vi "remove void rows.vi"(8 "error in":errorcluster, 11 "Group run list input":string[][](array[string])) -> (0 "error out":errorcluster, 3 "Group run list":string[][](array[string]))   [LabVIEW 2016]
doc: "This vi removes any empty spots from the run order."
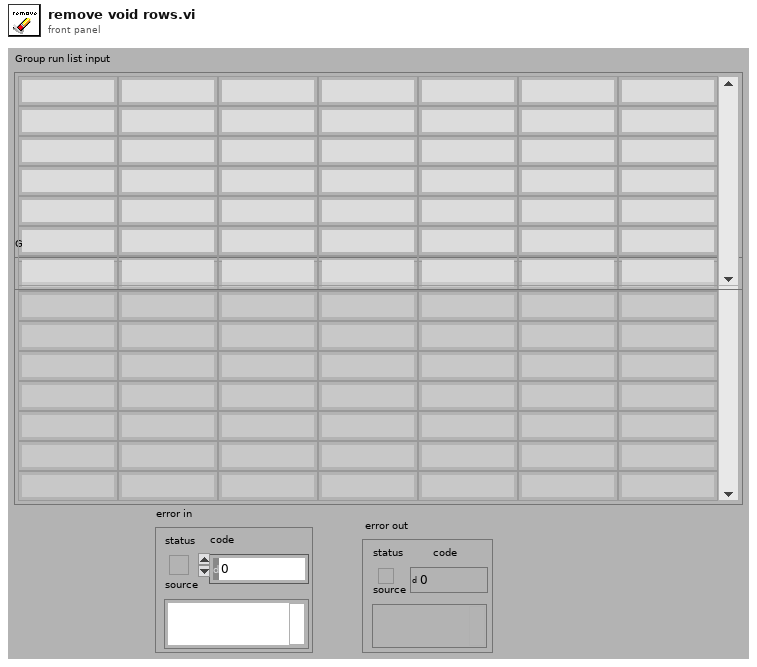
[diagram p1: front panel]
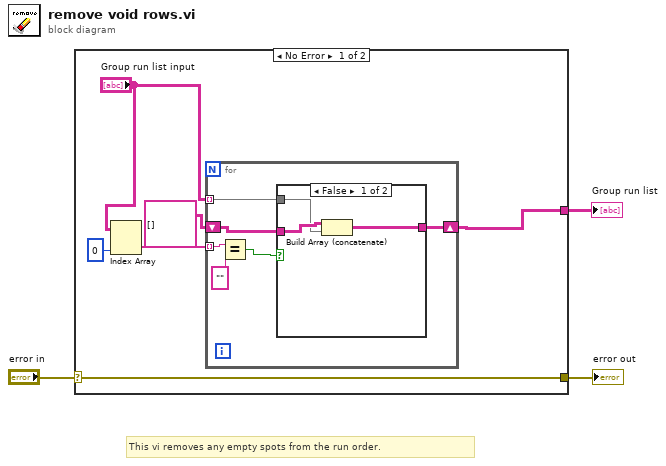
[diagram p0: block diagram]
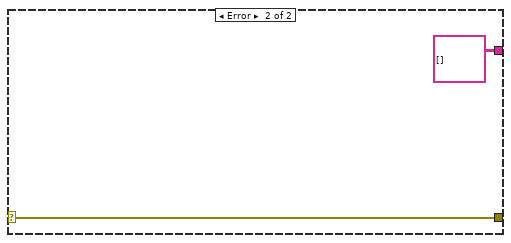
[diagram p3: hidden frame]
diagram:
  # "This vi removes any empty spots from the run order."
  n1 = case shown="No Error" "error in" {
    selector: "error in" -> [w4 w21]
    tunnel: [w5 string[][] []] -> w3
    tunnel: [w4 w21] -> w1
    frame No Error {
      n2 = Index Array(array="Group run list input", index (col)=0 ("disabled index (col)")) -> (element=w8:string[])  [unwired: 1 in]
      n3 = for {
        tunnel: w8 -> [w15] mode=indexing
        tunnel: "Group run list input" -> [w12] mode=indexing
        shift-right: [w11] -> w5
        shift-left: string[][] [] -> [w10]
        n4 = Equal?(x=w15, y="") -> (x = y?=w13:bool)
        n5 = case shown="False" w13 {
          tunnel: w12 -> [w16 _]
          tunnel: [w18 w19] -> w11
          tunnel: w10 -> [w17 w19]
          frame False {
            n6 = Build Array (concatenate)(w17, w16) -> (w18:string[][])
          }
          frame True {
          }
        }
      }
    }
    frame Error {
    }
  }
  "error out" <- w1
  "Group run list" <- w3
